vi "Lectrure 1 example 2.vi"() -> ()   [LabVIEW 2024]
panel:
  out "y":dbl
  in  "x":dbl
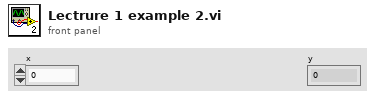
[diagram p1: front panel]
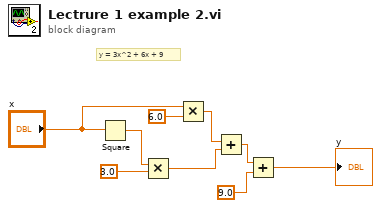
[diagram p0: block diagram]
diagram:
  # "y = 3x^2 + 6x + 9"
  n1 = Square(x="x") -> (x^2=w8:dbl)
  n2 = Multiply(x=w8, y=3.0) -> (x*y=w4:dbl)
  n3 = Multiply(x="x", y=6.0) -> (x*y=w5:dbl)
  n4 = Add(x=w5, y=w4) -> (x+y=w3:dbl)
  n5 = Add(x=w3, y=9.0) -> (x+y=→"y":dbl)
